vi "arrayMean.vi"(3 "Array":u16[][](array[numeric])) -> (0 "size":i32, 1 "mean":dbl)   [LabVIEW 2023]
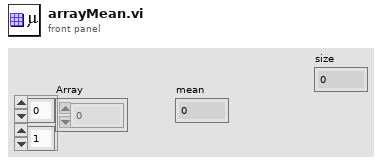
[diagram p1: front panel]
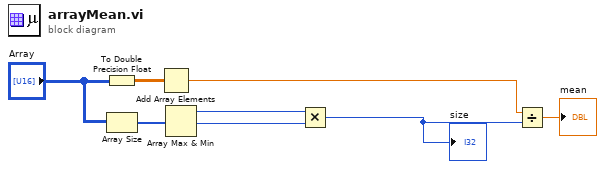
[diagram p0: block diagram]
diagram:
  n1 = To Double Precision Float(number="Array") -> (double precision float=w2:dbl[][])
  n2 = Array Size(array="Array") -> (size(s)=w1:i32[])
  n3 = Add Array Elements(numeric array=w2) -> (sum=w3:dbl)
  n4 = Array Max & Min(array=w1) -> (max value=w5:i32, min value=w6:i32)  [unwired: 2 out]
  n5 = Multiply(x=w5, y=w6) -> (x*y=w7:i32)
  "size" <- w7
  n6 = Divide(x=w3, y=w7) -> (x/y=→"mean":dbl)
